vi "Sync-Call with AdvanceAPI.vi"() -> ()   [LabVIEW 2020]
uses:
  <userlib>/_NEVSTOP/JKI State Machine++/JKI State Machine++.lvlib
panel:
  out "Arguments":string="DoA"
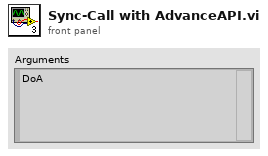
[diagram p1: front panel]
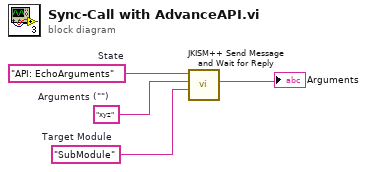
[diagram p0: block diagram]
diagram:
  w2 = "SubModule"  # Target Module
  w3 = "xyz"  # Arguments ("")
  w4 = "API: EchoArguments"  # State
  n1 = call <userlib>:"JKISM++ Send Message and Wait for Reply.vi"("Target Module"=w2, "Arguments (\"\")"=w3, "State"=w4) -> ("Arguments"=→"Arguments":string)  [unwired: 7 in, 1 out]
